vi "Query Method.vi"(8 "error in (no error)":errorcluster {"code" format="%.0x"}, 9 "RetValBufferSize":i32=2048 caption="RetValBufferSize (2048)", 11 "instrument handle":refnum<k15>) -> (0 "error out":errorcluster {"code" format="%.0x"}, 1 "RetValActualSize":i32, 2 "RetVal":i32[](array[numeric]), 3 "instrument handle out":refnum<k15>)   [LabVIEW 2009, in "Keysight XSAn.lvlib"]
doc: "Queries the carrier configuration method settings.\n\nSupported Models: M9290A, N8973B, N8974B, N8975B, N8976B, N9000A, N9000B, N9010A, N9010B, N9020A, N9020B, N9030A, N9030B, N9038A, N9040B, N9041B, SPN9003A, SPN9026A"
uses:
  <instrlib>/Keysight XSAn/Keysight XSAn.lvlib
  AgXSAn.dll
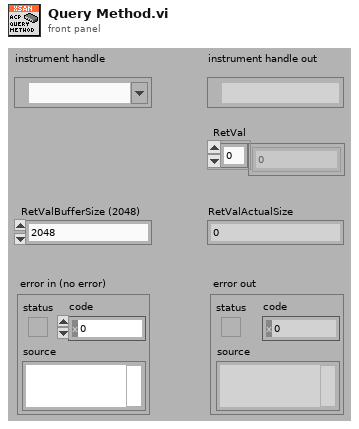
[diagram p1: front panel]
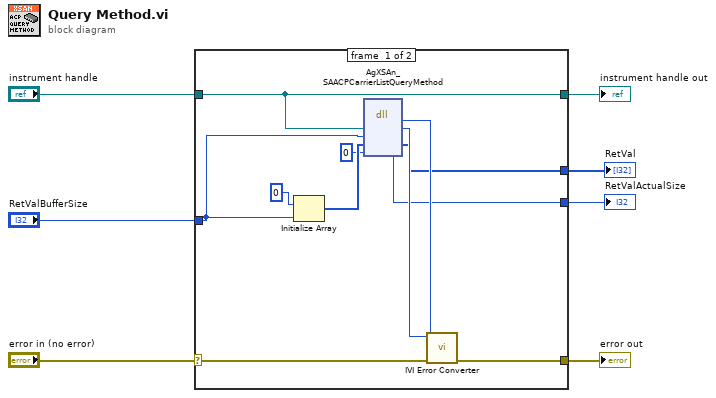
[diagram p0: block diagram]
diagram:
  n1 = case shown="No Error" "error in (no error)" {
    selector: "error in (no error)" -> [w16 w20]
    tunnel: [w15 w20] -> w7
    tunnel: "instrument handle" -> [w9 w19]
    tunnel: "RetValBufferSize" -> [w8 _]
    tunnel: [w12 _] -> w4
    tunnel: [w10 _] -> w3
    tunnel: [w9 w19] -> w1
    frame #0 {
      n2 = Initialize Array(0 ("element"), w8) -> (w14:i32[])
      n3 = dll-call lib="AgXSAn**.dll" fn="AgXSAn_SAACPCarrierListQueryMethod"("Vi"=w9, "RetValBufferSize"=w8, "RetVal"=w14, "RetValActualSize"=0) -> (w17:i32, "Vi"=w18:u32, "RetVal"=w12:i32[], "RetValActualSize"=w10:i32)  [unwired: 4 in, 2 out]
      n4 = call <instrlib>:"IVI Error Converter.vi"("error in (no error)"=w16, "IVI error code (0)"=w17, "instrument handle"=w18) -> ("error out"=w15:errorcluster)  [unwired: 7 in, 1 out]
    }
    frame #1 {
    }
  }
  "error out" <- w7
  "instrument handle out" <- w1
  "RetVal" <- w4
  "RetValActualSize" <- w3
